vi "Read Overlays cluster.vi"(8 "error in (no error)":errorcluster, 11 "Data in":refnum<class "Data.lvclass">) -> (0 "error out":errorcluster, 2 "Overlays cluster":T1, 3 "Data out":refnum<class "Data.lvclass">)   [LabVIEW 2018, in "Tracks Repair.lvlib" / "Data.lvclass"]
uses:
  Data.lvclass
  SubVi's/Controls/CTL_Overlays_cluster.ctl
  Data.lvclass/Data.ctl
  Common_Resources.lvlib
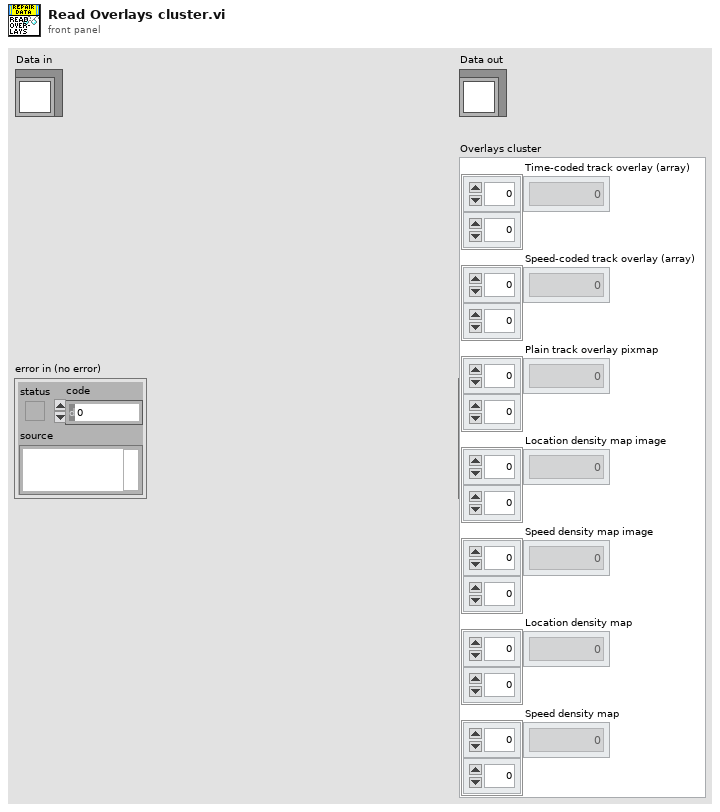
[diagram p1: front panel]
types:
  T1 = typedef "Common_Resources.lvlib/CTL_Overlays_cluster.ctl" = cluster{"Time-coded track overlay (array)":u32[][], "Speed-coded track overlay (array)":u32[][], "Plain track overlay pixmap":u32[][], "Location density map image":u32[][], "Speed density map image":u32[][], "Location density map":dbl[][], "Speed density map":dbl[][]}
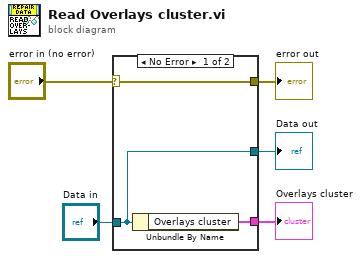
[diagram p0: block diagram]
diagram:
  n1 = case shown="No Error" "error in (no error)" {
    selector: "error in (no error)" -> [w8 w9]
    tunnel: [w8 w9] -> w4
    tunnel: [w7 w10] -> w2
    tunnel: "Data in" -> [w7 w10]
    tunnel: [w6 _] -> w1
    frame No Error {
      n2 = Unbundle By Name(w7) -> ("Overlays cluster"=w6:T1)
    }
    frame Error {
    }
  }
  "error out" <- w4
  "Data out" <- w2
  "Overlays cluster" <- w1
